vi "industrial project.vi"() -> ()   [LabVIEW 2018]
uses:
  Control 1.ctl
  Control 2.ctl
  Control 5.ctl
  <vilib>/DAQmx/read.llb/DAQmx Read (Analog DBL 1Chan 1Samp).vi
  <vilib>/DAQmx/create/channels.llb/DAQmx Create Channel (AI-Temperature-Thermocouple).vi
  <vilib>/DAQmx/configure/timing.llb/DAQmx Timing (Sample Clock).vi
  <vilib>/DAQmx/miscellaneous.llb/DAQmx Fill In Error Info.vi
  <vilib>/DAQmx/create/channels.llb/DAQmx Create Channel (AI-Voltage-Basic).vi
  <vilib>/DAQmx/create/channels.llb/DAQmx Create Channel (AI-Temperature-RTD).vi
panel:
  out "Thermometer":dbl(slide) scale=0.0..100.0
  out "Waveform Chart":dbl(graph)
  in  "Tab Control":enum32{"thermocouple", "RTD", "Thermistor"}(tab)
  in  "thermocouple type":i32(ring)=10072 items=["J"=10072, "K"=10073, "N"=10077, "R"=10082, "S"=10085, "T"=10086, "B"=10047, "E"=10055]
  in  "physical channels":T1
  in  "rate":dbl=1000.0 format="%0.2f"
  in  "sample mode":T2=10178 items=["Finite Samples"=10178, "Continuous Samples"=10123, "Hardware Timed Single Point"=12522]
  in  "stop":bool
  in  "physical channels RTD":T3
  in  "rateRTD":dbl=1000.0 format="%0.2f"
  in  "rtd type":i32(ring)=12481 items=["Pt3750"=12481, "Pt3851"=10071, "Pt3911"=12482, "Pt3916"=10069, "Pt3920"=10053, "Pt3928"=12483, "Custom"=10137]
  in  "stop 2":bool
  in  "sample mode RTD":i32(ring)=10178 items=["Finite Samples"=10178, "Continuous Samples"=10123, "Hardware Timed Single Point"=12522]
  in  "physical channels 2":tag
  in  "rate 2":dbl=1000.0 format="%0.2f"
  in  "sample mode 2":i32(ring)=10178 items=["Finite Samples"=10178, "Continuous Samples"=10123, "Hardware Timed Single Point"=12522]
  in  "stop 3":bool
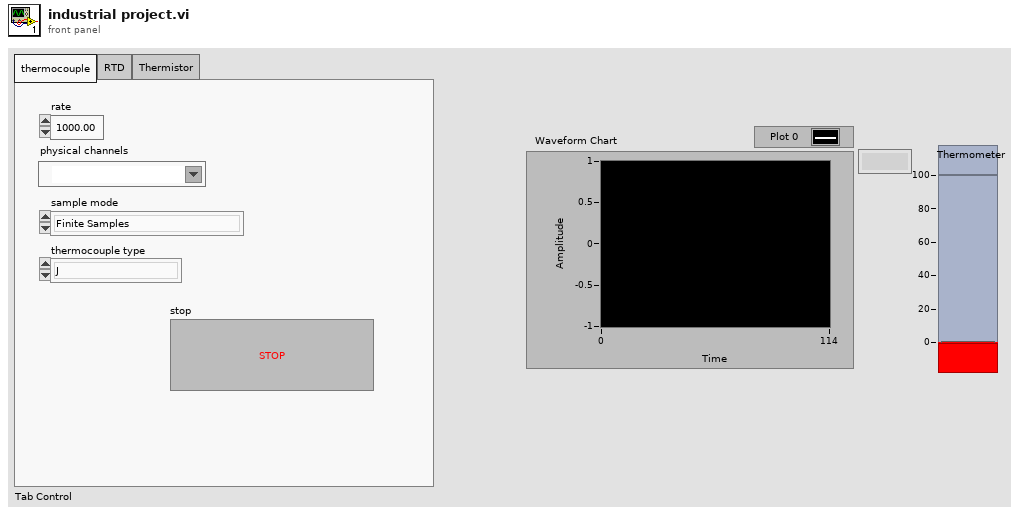
[diagram p1: front panel]
types:
  T1 = typedef "Control 1.ctl" = tag
  T2 = typedef "Control 2.ctl" = i32
  T3 = typedef "Control 5.ctl" = tag
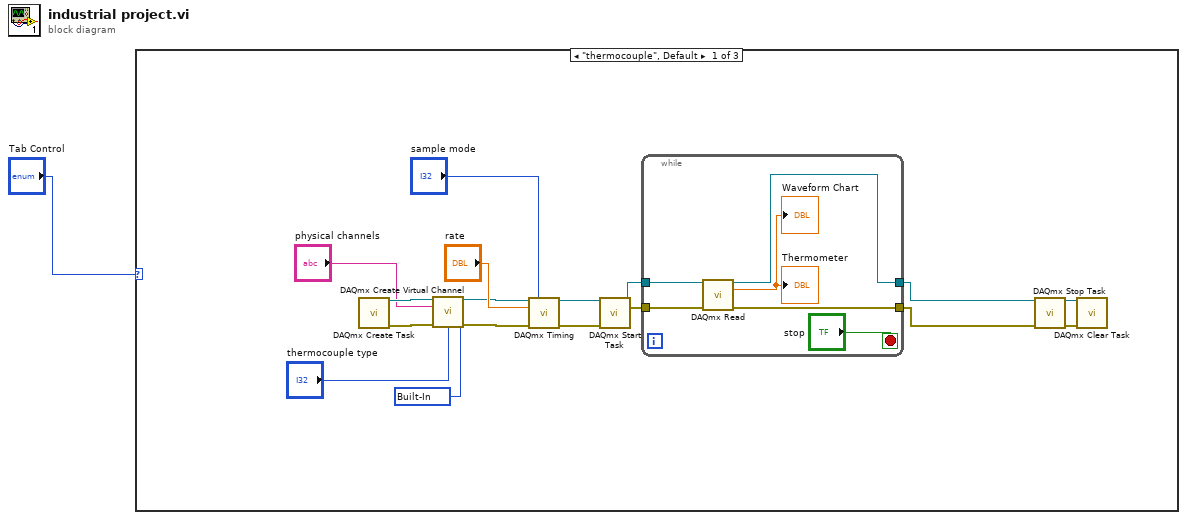
[diagram p0: block diagram]
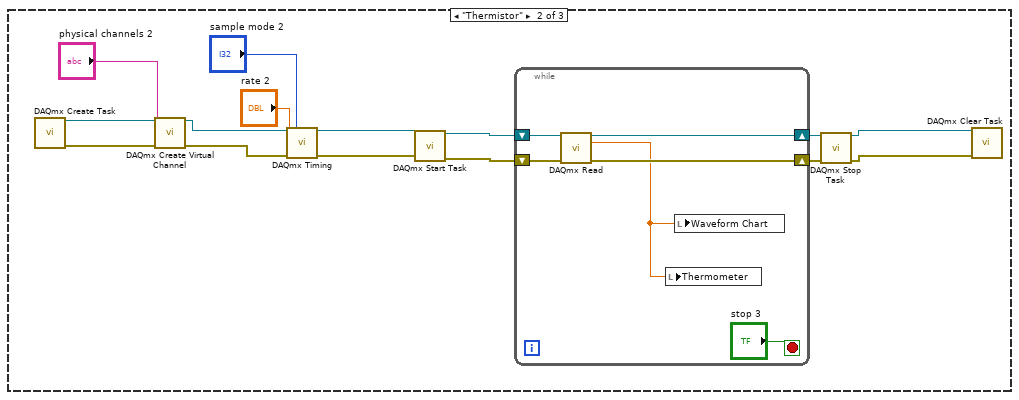
[diagram p2: hidden frame]
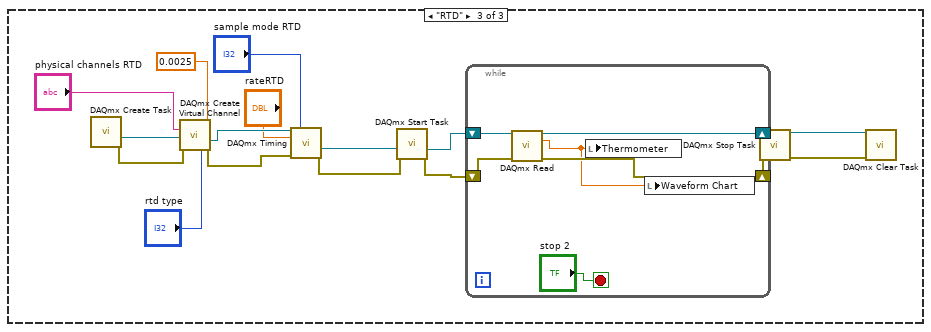
[diagram p3: hidden frame]
diagram:
  n1 = case shown="\"thermocouple\", Default" "Tab Control" {
    frame "thermocouple", Default {
      w2 = 10200 items=["Built-In"=10200, "Constant Value"=10116, "Channel"=10113] ("cjc source")
      n2 = call <vilib>:"DAQmx Create Task.vi"() -> ("task out"=w18:refnum<k21>, "error out"=w12:errorcluster)  [unwired: 14 in]
      n3 = call-poly <vilib>:"DAQmx Create Virtual Channel.vi"("task in"=w18, "physical channels"="physical channels", "cjc source"=w2, "error in"=w12, "thermocouple type"="thermocouple type") -> ("task out"=w14:refnum<k21>, "error out"=w13:errorcluster)  [unwired: 9 in]
      n4 = call-poly <vilib>:"DAQmx Timing.vi"("task/channels in"=w14, "sample mode"="sample mode", "rate"="rate", "error in"=w13) -> ("task out"=w10:refnum<k21>, "error out"=w9:errorcluster)  [unwired: 10 in]
      n5 = call <vilib>:"DAQmx Start Task.vi"("task/channels in"=w10, "error in"=w9) -> ("task out"=w8:refnum<k21>, "error out"=w7:errorcluster)  [unwired: 12 in]
      n6 = while {
        tunnel: w8 -> [w24]
        tunnel: w7 -> [w23]
        tunnel: [w22] -> w6
        tunnel: [w21] -> w5
        stop <- "stop" stop-if-true
        n7 = call-poly <vilib>:"DAQmx Read.vi"("task/channels in"=w24, "error in"=w23) -> ("task out"=w22:refnum<k21>, "data"=→"Waveform Chart" →"Thermometer":dbl, "error out"=w21:errorcluster)  [unwired: 11 in]
      }
      n8 = call <vilib>:"DAQmx Stop Task.vi"("task/channels in"=w6, "error in"=w5) -> ("task out"=w4:refnum<k21>, "error out"=w3:errorcluster)  [unwired: 12 in]
      n9 = call <vilib>:"DAQmx Clear Task.vi"("task in"=w4, "error in"=w3) -> ()  [unwired: 13 in, 1 out]
    }
    frame "Thermistor" {
      n10 = call <vilib>:"DAQmx Create Task.vi"() -> ("task out"=w39:refnum<k21>, "error out"=w33:errorcluster)  [unwired: 14 in]
      n11 = call-poly <vilib>:"DAQmx Create Virtual Channel.vi"("task in"=w39, "physical channels"="physical channels 2", "error in"=w33) -> ("task out"=w38:refnum<k21>, "error out"=w32:errorcluster)  [unwired: 11 in]
      n12 = call-poly <vilib>:"DAQmx Timing.vi"("task/channels in"=w38, "sample mode"="sample mode 2", "rate"="rate 2", "error in"=w32) -> ("task out"=w37:refnum<k21>, "error out"=w31:errorcluster)  [unwired: 10 in]
      n13 = call <vilib>:"DAQmx Start Task.vi"("task/channels in"=w37, "error in"=w31) -> ("task out"=w36:refnum<k21>, "error out"=w30:errorcluster)  [unwired: 12 in]
      n14 = while {
        shift-right: [w44] -> w35
        shift-left: w36 -> [w45]
        shift-right: [w42] -> w29
        shift-left: w30 -> [w43]
        stop <- "stop 3" stop-if-true
        n15 = call-poly <vilib>:"DAQmx Read.vi"("task/channels in"=w45, "error in"=w43) -> ("task out"=w44:refnum<k21>, "data"=w41:dbl, "error out"=w42:errorcluster)  [unwired: 11 in]
        n16 = local write "Thermometer"(w41) -> ()
        n17 = local write "Waveform Chart"(w41) -> ()
      }
      n18 = call <vilib>:"DAQmx Stop Task.vi"("task/channels in"=w35, "error in"=w29) -> ("task out"=w34:refnum<k21>, "error out"=w28:errorcluster)  [unwired: 12 in]
      n19 = call <vilib>:"DAQmx Clear Task.vi"("task in"=w34, "error in"=w28) -> ()  [unwired: 13 in, 1 out]
    }
    frame "RTD" {
      n20 = call <vilib>:"DAQmx Create Task.vi"() -> ("task out"=w62:refnum<k21>, "error out"=w56:errorcluster)  [unwired: 14 in]
      n21 = call-poly <vilib>:"DAQmx Create Virtual Channel.vi"("task in"=w62, "physical channels"="physical channels RTD", "current excitation value"=0.0025, "error in"=w56, "rtd type"="rtd type") -> ("task out"=w61:refnum<k21>, "error out"=w55:errorcluster)  [unwired: 9 in]
      n22 = call-poly <vilib>:"DAQmx Timing.vi"("task/channels in"=w61, "sample mode"="sample mode RTD", "rate"="rateRTD", "error in"=w55) -> ("task out"=w60:refnum<k21>, "error out"=w54:errorcluster)  [unwired: 10 in]
      n23 = call <vilib>:"DAQmx Start Task.vi"("task/channels in"=w60, "error in"=w54) -> ("task out"=w59:refnum<k21>, "error out"=w53:errorcluster)  [unwired: 12 in]
      n24 = while {
        shift-right: [w67] -> w58
        shift-left: w59 -> [w68]
        shift-right: [w65] -> w52
        shift-left: w53 -> [w66]
        stop <- "stop 2" stop-if-true
        n25 = call-poly <vilib>:"DAQmx Read.vi"("task/channels in"=w68, "error in"=w66) -> ("task out"=w67:refnum<k21>, "data"=w63:dbl, "error out"=w65:errorcluster)  [unwired: 11 in]
        n26 = local write "Thermometer"(w63) -> ()
        n27 = local write "Waveform Chart"(w63) -> ()
      }
      n28 = call <vilib>:"DAQmx Stop Task.vi"("task/channels in"=w58, "error in"=w52) -> ("task out"=w57:refnum<k21>, "error out"=w51:errorcluster)  [unwired: 12 in]
      n29 = call <vilib>:"DAQmx Clear Task.vi"("task in"=w57, "error in"=w51) -> ()  [unwired: 13 in, 1 out]
    }
  }
